vi "Colleague_Create.vi"(8 "Error In":errorcluster, 10 "Mediator":refnum<class "Mediator.lvclass">, 11 "reference in":refnum<class "Colleague.lvclass">) -> (0 "Error Out":errorcluster, 3 "reference out":refnum<class "Colleague.lvclass">)   [LabVIEW 2020, in "Colleague.lvclass"]
uses:
  Colleague.lvclass
  Mediator_class/Mediator.lvclass
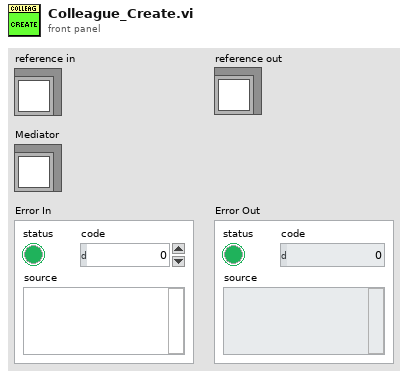
[diagram p1: front panel]
types:
  T1 = typedef "Colleague.lvclass/ObjectAttributes.ctl" = cluster{"Mediator":refnum<class "Mediator.lvclass">}
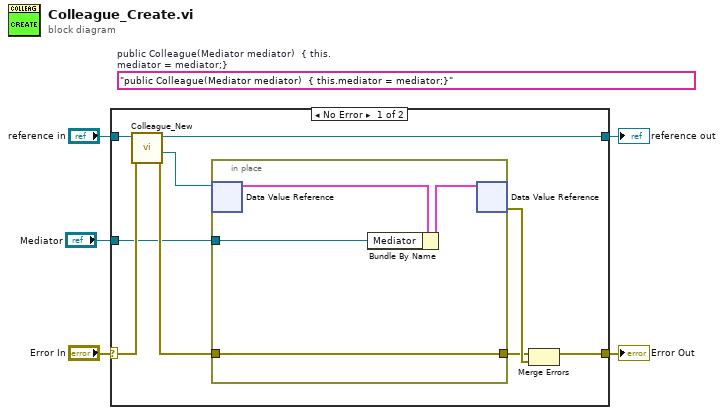
[diagram p0: block diagram]
diagram:
  (unwired) "public Colleague(Mediator mediator)  { this.mediator = mediator;}"  # public Colleague(Mediator mediator)  { this.mediator = mediator;}
  n1 = case shown="No Error" "Error In" {
    selector: "Error In" -> [w13 w20]
    tunnel: [w7 w20] -> w4
    tunnel: "reference in" -> [w14 w19]
    tunnel: [w12 w19] -> w2
    tunnel: "Mediator" -> [w6 _]
    frame No Error {
      n2 = call "Colleague_New.vi"("error in (no error)"=w13, "reference in"=w14) -> ("error out"=w9:errorcluster, "DVRRefOut"=w10:refnum<data-value>, "reference out"=w12:refnum<class "Colleague.lvclass">)  [unwired: 6 in, 1 out]
      n3 = in-place {
        in-place-border: w9 -> [w16]
        in-place-border: [w16] -> w8
        in-place-border: w6 -> [w15]
        n4 = in-place-dvr #1(w10) -> (w17:T1)  [unwired: 1 out]
        n5 = Bundle By Name(cluster=w17, "Mediator"=w15) -> (w18:T1)
        n6 = in-place-dvr #1(w18) -> (w11:errorcluster)  [unwired: 1 out]
      }
      n7 = Merge Errors(w8, w11) -> (w7:errorcluster)
    }
    frame Error {
      # "VI-TechBaseTemplate_Simple_4x4x4"
    }
  }
  "Error Out" <- w4
  "reference out" <- w2
